vi "Cleanup.vi"(8 "error in (no error)":errorcluster, 11 "Action in":refnum<class "Action.lvclass">) -> (0 "error out":errorcluster, 3 "Action out":refnum<class "Action.lvclass">)   [LabVIEW 2020, in "neg-pkg.lvlib" / "Action.lvclass"]
uses:
  Action.lvclass
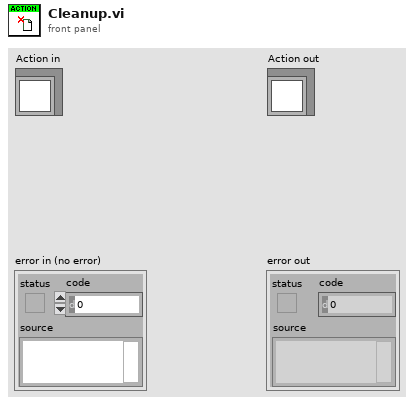
[diagram p1: front panel]
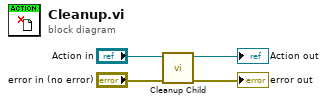
[diagram p0: block diagram]
diagram:
  n1 = call-dynamic "Cleanup Child.vi"("error in (no error)"="error in (no error)", "Action in"="Action in") -> ("error out"=→"error out":errorcluster, "Action out"=→"Action out":refnum<class "Action.lvclass">)  [unwired: 8 in]
